vi "Actor Destroy.vi"(11 "Dev Actor in":refnum<class "Dev Actor.lvclass">) -> (0 "error out":errorcluster, 3 "Dev Actor out":refnum<class "Dev Actor.lvclass">)   [LabVIEW 2021, in "Dev Actor.lvlib" / "Dev Actor.lvclass"]
uses:
  Dev Actor.lvclass
  Dev Actor.lvclass/Dev Actor.ctl
  LVCAM/LVCAM/Actor/Actor.lvclass
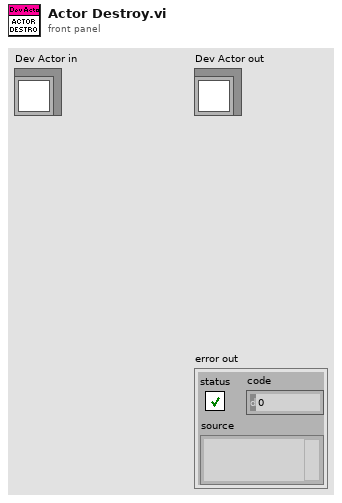
[diagram p1: front panel]
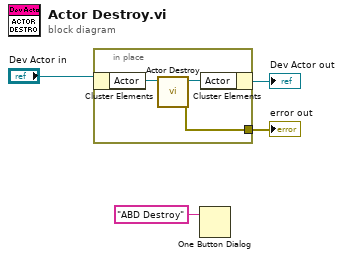
[diagram p0: block diagram]
diagram:
  n1 = in-place {
    in-place-border: [w5] -> w4
    n2 = in-place-cluster #1("Dev Actor in") -> ("Actor"=w7:refnum<class "Actor.lvclass">)
    n3 = call-dynamic "Actor Destroy.vi"("Actor Destroy in"=w7) -> ("error out"=w5:errorcluster, "Actor Destroy out"=w6:refnum<class "Actor.lvclass">)  [unwired: 9 in]
    n4 = in-place-cluster #1("Actor"=w6) -> (→"Dev Actor out":refnum<class "Dev Actor.lvclass">)
  }
  "error out" <- w4
  n5 = One Button Dialog(message="ABD Destroy") -> ()  [unwired: 1 in, 1 out]
